vi "Rapid Filtration Controller_ver1.1 (2).vi"() -> ()   [LabVIEW 2010]
uses:
  <vilib>/Instr/_visa.llb/VISA Configure Serial Port (Instr).vi
panel:
  in  "Port Connection":refnum<visa-resource-name>
  out "Run Status":bool
  out "Pump Position":bool
  out "?":string
  out "Connection status":bool
  in  "stop":bool
  out "read buffer":string
  out "error out 2":errorcluster
  in  "Tab Control":enum32{"Run Mode", "Calibration"}(tab)
  in  "Flow Rate (ml/s)":dbl(slide)=0.15 min=0.15 max=9.0 scale=0.1..9.0 scale format="%#_2f"
  in  "Time (ms)":dbl=50.0 min=10.0 max=9000.0 step=1.0
  in  "Run":bool
  out "Pulse out":u16
  in  "Max Flow Rate":dbl=9.0
  in  "Min Flow Rate":dbl=0.15
  in  "Max Freq":dbl=2017.0
  in  "Min Freq":dbl=45.0
  in  "Time (ms)":dbl=50.0 min=10.0 max=9000.0 step=1.0
  in  "Pump":bool
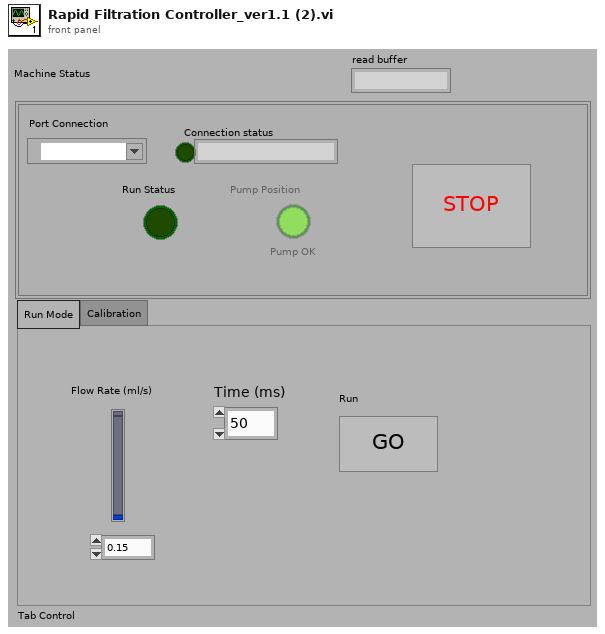
[diagram p1: front panel]
types:
  T1 = enum8{"Enabled", "Disabled", "Disabled and Grayed Out"}
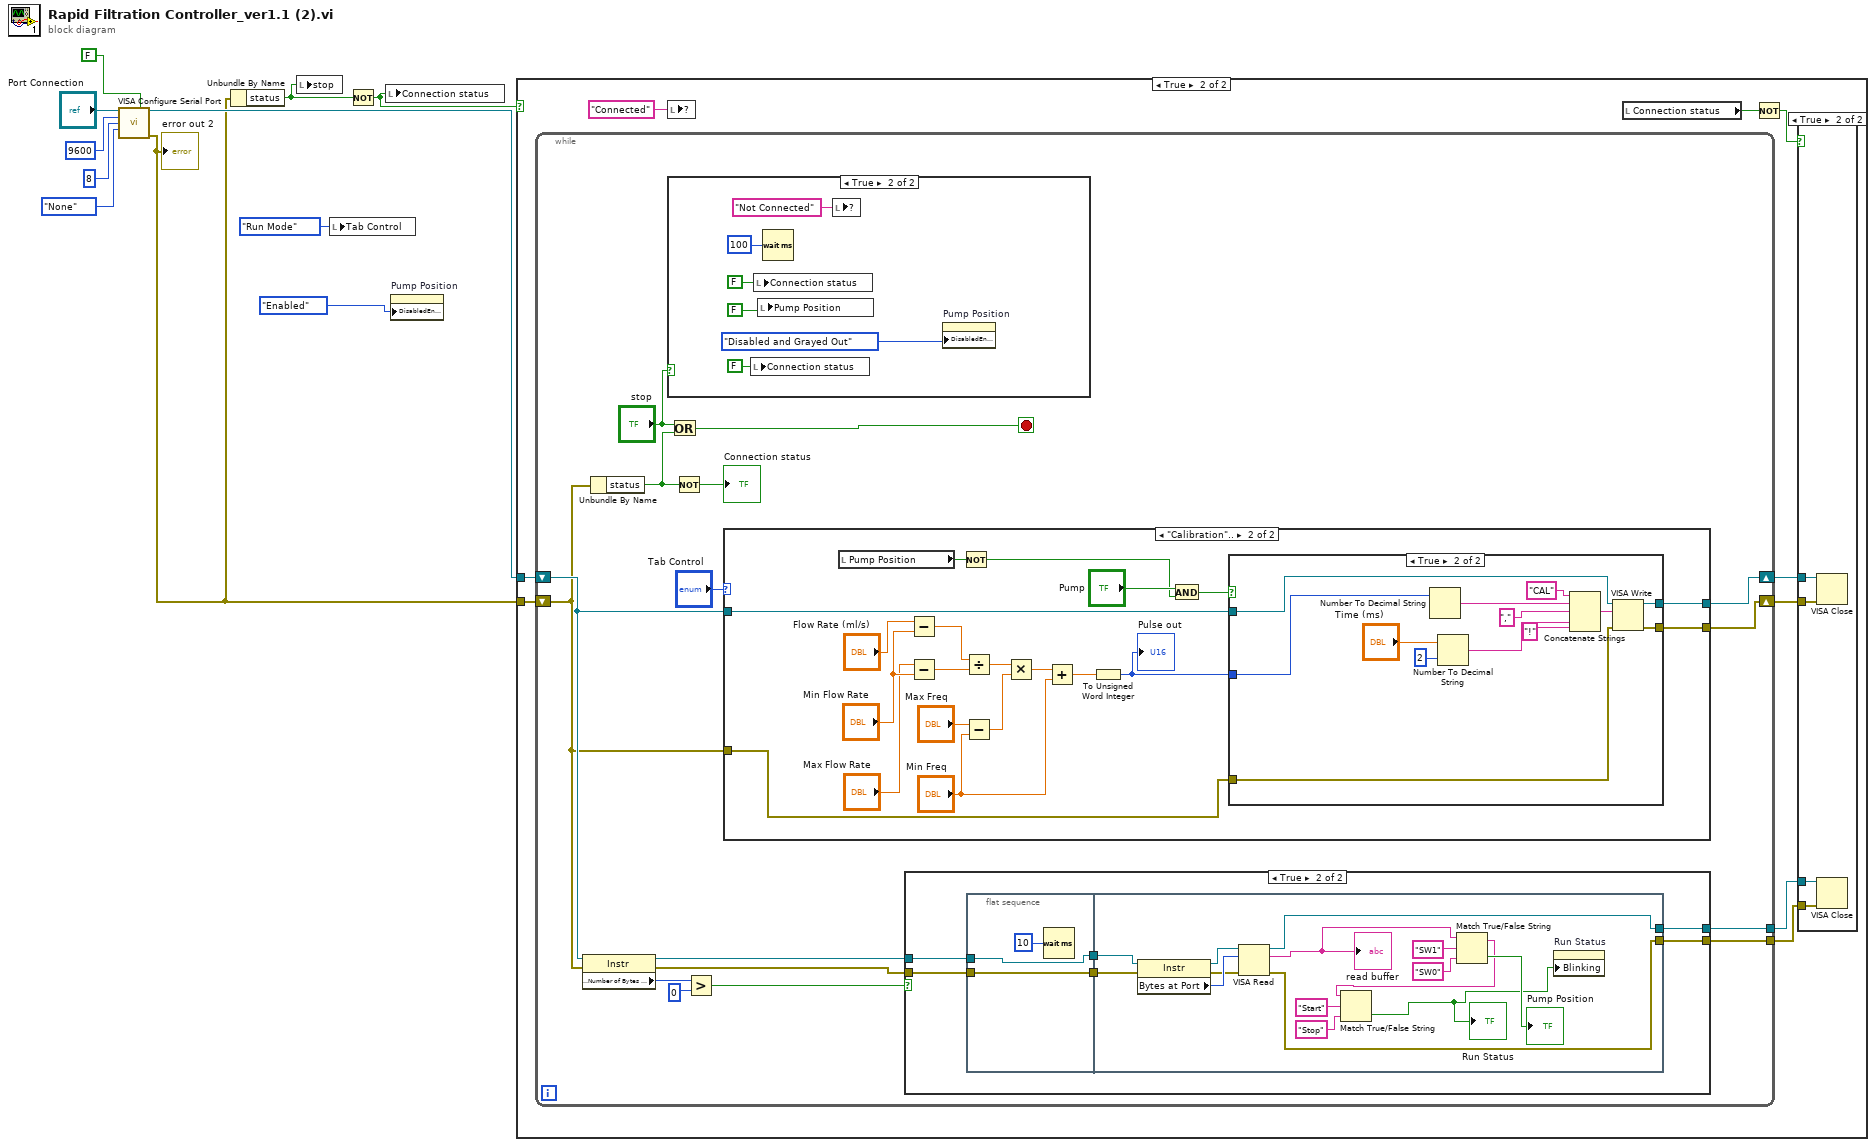
[diagram p0: block diagram]
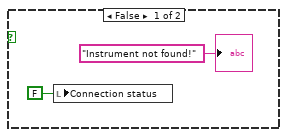
[diagram p2: hidden frame]
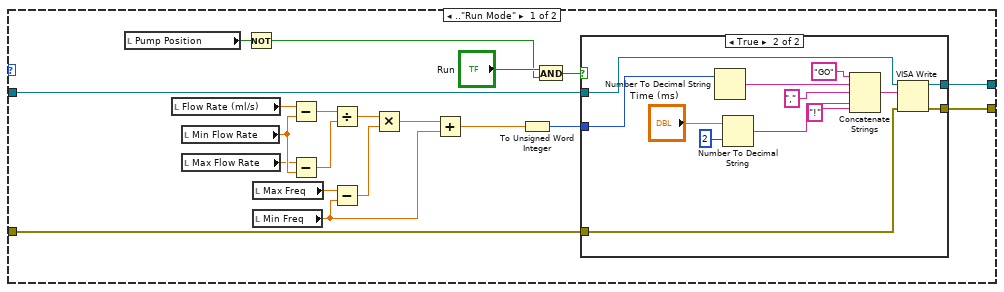
[diagram p4: hidden frame]
diagram:
  n1 = call-poly "VISA Configure Serial Port"("VISA resource name"="Port Connection", "Enable Termination\nChar (T)"=FALSE ("Enable Termination\nChar (T)"), "baud rate (9600)"=u32 9600, "data bits (8)"=u16 8, "parity (0:none)"=enum16{"None", "Odd", "Even", "Mark", "Space"}."None") -> ("VISA resource name out"=w7:refnum<visa-resource-name>, "error out"=w6:errorcluster)  [unwired: 9 in]
  "error out 2" <- w6
  n2 = Unbundle By Name(w6) -> ("status"=w5:bool)
  n3 = local write "stop"(w5) -> ()
  n4 = local write "Tab Control"(enum32{"Run Mode", "Calibration"}."Run Mode" ("Tab Control")) -> ()
  n5 = Not(x=w5) -> (.not. x?=w3:bool)
  n6 = local write "Connection status"(w3) -> ()
  n7 = property on="Pump Position" class="Bool (strict)"("DisabledEnum"=T1."Enabled" ("Disabled")) -> ()  [unwired: 2 in, 2 out]
  n8 = case shown="True" w3 {
    tunnel: w7 -> [_ w22]
    tunnel: w6 -> [_ w17]
    frame False {
      n9 = local write "Connection status"(FALSE ("Connection status")) -> ()
      "?" <- "Instrument not found!"
    }
    frame True {
      n10 = while {
        tunnel: [w35] -> w20
        tunnel: [w33] -> w19
        shift-right: [w39] -> w21
        shift-left: w17 -> [w30]
        shift-right: [w34] -> w18
        shift-left: w22 -> [w40]
        stop <- w32 stop-if-true
        n11 = property class="Instr"(reference=w40, error in=w30) -> (reference out=w38:refnum<visa-resource-name>, error out=w37:errorcluster, "Serial Settings:Number of Bytes at Serial Port"=w41:u32)
        n12 = Unbundle By Name(w30) -> ("status"=w31:bool)
        n13 = case shown="True" "stop" {
          frame False {
          }
          frame True {
            n14 = local write "Connection status"(FALSE ("Run Status")) -> ()
            n15 = local write "Connection status"(FALSE ("Connection status")) -> ()
            n16 = local write "Pump Position"(FALSE ("Pump Position")) -> ()
            n17 = Wait (ms)(milliseconds to wait=u32 100) -> ()  [unwired: 1 out]
            n18 = local write item#12("Not Connected") -> ()
            n19 = property on="Pump Position" class="Bool (strict)"("DisabledEnum"=T1."Disabled and Grayed Out" ("Disabled")) -> ()  [unwired: 2 in, 2 out]
          }
        }
        n20 = Or(x="stop", y=w31) -> (x .or. y?=w32:bool)
        n21 = Not(x=w31) -> (.not. x?=→"Connection status":bool)
        n22 = Greater?(x=w41, y=u32 0) -> (0:w36:bool)
        n23 = case shown="\"Calibration\".." "Tab Control" {
          tunnel: w40 -> [w60 w86]
          tunnel: [w59 w89] -> w39
          tunnel: [w52 w88] -> w34
          tunnel: w30 -> [w51 w87]
          frame .."Run Mode" {
            n24 = local read "Pump Position"() -> (w58:bool)
            n25 = local read "Flow Rate (ml/s)"() -> (w48:dbl)
            n26 = local read "Min Flow Rate"() -> (w47:dbl)
            n27 = local read "Max Flow Rate"() -> (w45:dbl)
            n28 = Not(x=w58) -> (.not. x?=w43:bool)
            n29 = local read "Max Freq"() -> (w46:dbl)
            n30 = local read "Min Freq"() -> (w44:dbl)
            n31 = Subtract(x=w48, y=w47) -> (x-y=w53:dbl)
            n32 = Subtract(x=w45, y=w47) -> (x-y=w54:dbl)
            n33 = Divide(x=w53, y=w54) -> (x/y=w55:dbl)
            n34 = Subtract(x=w46, y=w44) -> (x-y=w56:dbl)
            n35 = Multiply(x=w55, y=w56) -> (x*y=w57:dbl)
            n36 = Add(x=w57, y=w44) -> (x+y=w50:dbl)
            n37 = To Unsigned Word Integer(number=w50) -> (unsigned 16bit integer=w49:u16)
            n38 = And(x="Run", y=w43) -> (x .and. y?=w61:bool)
            n39 = case shown="True" w61 {
              tunnel: w60 -> [w64 w77]
              tunnel: w51 -> [w63 w76]
              tunnel: [w64 w69] -> w52
              tunnel: [w63 w68] -> w59
              tunnel: w49 -> [_ w65]
              frame False {
              }
              frame True {
                n40 = Number To Decimal String(number=w65) -> (decimal integer string=w74:string)  [unwired: 1 in]
                n41 = Number To Decimal String(number="Time (ms)", width (-)=i16 2) -> (decimal integer string=w71:string)
                n42 = Concatenate Strings("GO", w74, "," ("string"), w71, "!" ("string")) -> (w70:string)
                n43 = VISA Write(VISA resource name=w77, write buffer=w70, error in (no error)=w76) -> (VISA resource name out=w69:refnum<visa-resource-name>, error out=w68:errorcluster)  [unwired: 1 out]
              }
            }
          }
          frame "Calibration".. {
            n44 = local read "Pump Position"() -> (w96:bool)
            n45 = Subtract(x="Flow Rate (ml/s)", y="Min Flow Rate") -> (x-y=w91:dbl)
            n46 = Subtract(x="Max Flow Rate", y="Min Flow Rate") -> (x-y=w92:dbl)
            n47 = Not(x=w96) -> (.not. x?=w78:bool)
            n48 = Divide(x=w91, y=w92) -> (x/y=w93:dbl)
            n49 = Subtract(x="Max Freq", y="Min Freq") -> (x-y=w94:dbl)
            n50 = Multiply(x=w93, y=w94) -> (x*y=w95:dbl)
            n51 = Add(x=w95, y="Min Freq") -> (x+y=w90:dbl)
            n52 = To Unsigned Word Integer(number=w90) -> (unsigned 16bit integer=w79:u16)
            "Pulse out" <- w79
            n53 = And(x="Pump", y=w78) -> (x .and. y?=w80:bool)
            n54 = case shown="True" w80 {
              tunnel: [w98 w104] -> w89
              tunnel: [w99 w103] -> w88
              tunnel: w87 -> [w98 w102]
              tunnel: w86 -> [w99 w101]
              tunnel: w79 -> [_ w100]
              frame False {
              }
              frame True {
                n55 = Number To Decimal String(number=w100) -> (decimal integer string=w111:string)  [unwired: 1 in]
                n56 = Number To Decimal String(number="Time (ms)", width (-)=i16 2) -> (decimal integer string=w108:string)
                n57 = Concatenate Strings("CAL", w111, "," ("string"), w108, "!" ("string")) -> (w107:string)
                n58 = VISA Write(VISA resource name=w101, write buffer=w107, error in (no error)=w102) -> (VISA resource name out=w103:refnum<visa-resource-name>, error out=w104:errorcluster)  [unwired: 1 out]
              }
            }
          }
        }
        n59 = case shown="True" w36 {
          tunnel: [w119 w123] -> w33
          tunnel: [w120 w124] -> w35
          tunnel: w38 -> [w120 w126]
          tunnel: w37 -> [w119 w125]
          frame False {
          }
          frame True {
            n60 = flat-sequence {
              tunnel: w125 -> [w128]
              tunnel: w126 -> [w129]
              tunnel: [w129] -> w122
              tunnel: [w128] -> w121
              tunnel: [w139] -> w124
              tunnel: [w138] -> w123
              tunnel: w122 -> [w141]
              tunnel: w121 -> [w140]
              frame #0 {
                n61 = Wait (ms)(milliseconds to wait=u32 10) -> ()  [unwired: 1 out]
              }
              frame #1 {
                n62 = property class="Instr"(reference=w141, error in=w140) -> (reference out=w143:refnum<visa-resource-name>, error out=w142:errorcluster, "Bytes at Port"=w144:u32)
                n63 = VISA Read(VISA resource name=w143, byte count=w144, error in (no error)=w142) -> (VISA resource name out=w139:refnum<visa-resource-name>, read buffer=w132:string, error out=w138:errorcluster)  [unwired: 1 out]
                "read buffer" <- w132
                n64 = Match True/False String(2:"SW0" ("false string"), 3:"SW1" ("true string"), 4:w132) -> (0:→"Pump Position":bool, 1:w131:string)
                n65 = Match True/False String(2:"Stop" ("false string"), 3:"Start" ("true string"), 4:w131) -> (0:w130:bool)  [unwired: 1 out]
                "Run Status" <- w130
                n66 = property on="Run Status" class="Bool (strict)"("Blinking"=w130) -> ()  [unwired: 2 in, 2 out]
              }
            }
          }
        }
      }
      n67 = local write item#12("Connected") -> ()
      n68 = local read "Connection status"() -> (w15:bool)
      n69 = Not(x=w15) -> (.not. x?=w14:bool)
      n70 = case shown="True" w14 {
        tunnel: w21 -> [_ w26]
        tunnel: w20 -> [_ w25]
        tunnel: w19 -> [_ w24]
        tunnel: w18 -> [_ w23]
        frame False {
        }
        frame True {
          n71 = VISA Close(VISA resource name=w23, error in (no error)=w26) -> ()  [unwired: 1 out]
          n72 = VISA Close(VISA resource name=w25, error in (no error)=w24) -> ()  [unwired: 1 out]
        }
      }
    }
  }
